vi "Robot Global Data.vi"() -> ()   [LabVIEW 2016]
doc: "This global VI can contain as many global variables as you need. Place a control on the panel, give it a good name. To read or write to it from a VI, drag the icon to the diagram of that VI. You can also drag from the project. Click on the node to change which global you access. You shouldn't have multiple locations writing to a global or it will cause a race-condition."
uses:
  <vilib>/Rock Robotics/WPI/Camera/WPI_CameraImageSize.ctl
  <vilib>/Rock Robotics/WPI/DriverStation/WPI_DriverStationRobotMode2.ctl
panel:
  out "Vision Nothing In Sight":bool
  in  "Autonoums Delay":dbl
  in  "Vision align Range correction VARIABLE":dbl
  in  "Vision align Oscillation correction VARIABLE":dbl
  in  "Autonomos Gyro forward SPEED VARIABLE":dbl
  in  "Periodic Gyro forward SPEED VARIABLE":dbl
  in  "Accelerometer Z Axis":dbl
  in  "Accelerometer Y Axis":dbl
  in  "Accelerometer X Axis":dbl
  out "Gyro Rest?":bool
  in  "LEFT SPEED VARIABLE":dbl
  out "Autonomous Operating":bool
  out "Vision needed":bool
  in  "RIGHT SPEED VARIABLE":dbl
  in  "ClimbMotors":dbl
  in  "Enum Teleop Control":u16
  in  "Enum Teleop":T1(ring)
  out "Teleop Operating":bool
  in  "String Teleop":string
  in  "Motor Array":dbl[](array[numeric])
  out "Vision Enabled":bool
  out "auto proceed":bool
  in  "Vision Turn":dbl
  in  "LeftMotors":dbl
  in  "RightMotors":dbl
  in  "X?":dbl
  out "In range?":bool
  out "Logitech Right 9":bool
  out "Logitech Left 9":bool
  out "Logitech Right 7":bool
  out "Logitech Right 5":bool
  out "Logitech Right 6":bool
  out "Logitech Right 8":bool
  out "Logitech Right 4":bool
  out "Logitech Right 3":bool
  out "Logitech Right 2":bool
  out "Logitech Right 1":bool
  out "Logitech Left 7":bool
  out "Logitech Left 5":bool
  out "Logitech Left 6":bool
  out "Logitech Left 8":bool
  out "Logitech Left 4":bool
  out "Logitech Left 3":bool
  out "Logitech Left 2":bool
  out "Logitech Left 1":bool
  in  "Logitech Right Slider":dbl
  in  "Logitech Right Z axis":dbl
  in  "Logitech Right Y axis":dbl
  in  "Logitech Right X axis":dbl
  in  "Logitech Left Slider":dbl
  in  "Logitech Left Z axis":dbl
  in  "Logitech Left Y axis":dbl
  in  "Logitech Left X axis":dbl
  out "Xbox Left Joystick Button":bool
  out "Xbox Back":bool
  out "Xbox LB":bool
  out "Xbox RB":bool
  out "Xbox Start":bool
  out "Xbox Y":bool
  out "Xbox X":bool
  out "Xbox B":bool
  out "Xbox A":bool
  in  "Xbox Left Trigger":dbl
  in  "Xbox Right Trigger":dbl
  in  "Xbox Right X axis":dbl
  in  "Xbox Right Y axis":dbl
  in  "Xbox Left X axis":dbl
  in  "Xbox Left Y axis":dbl
  in  "TopRightMotor":dbl
  in  "TopLeftMotor":dbl
  in  "GyroAngularRate":dbl
  in  "GyroAngle":dbl
  in  "Robot Mode":T2
  in  "image size":T3=enum."320x240"
  in  "Enable Vision":bool
  # "Power To Motors :"
  # "Accelerometer Axis Data"
  # "DASHBOARD VARIABLES"
  # "Vsion processing things"
  # "Motor Oversight"
  # "Turns on when Teleop is active"
  # "Gyro Data"
  # "Turns on when Autonomos is active"
  # "Logitech Joystick Right"
  # "Logitech Joystick Left"
  # "Xbox Controls :"
  # "Teleop controls"
  # "Dunno wut dis is"
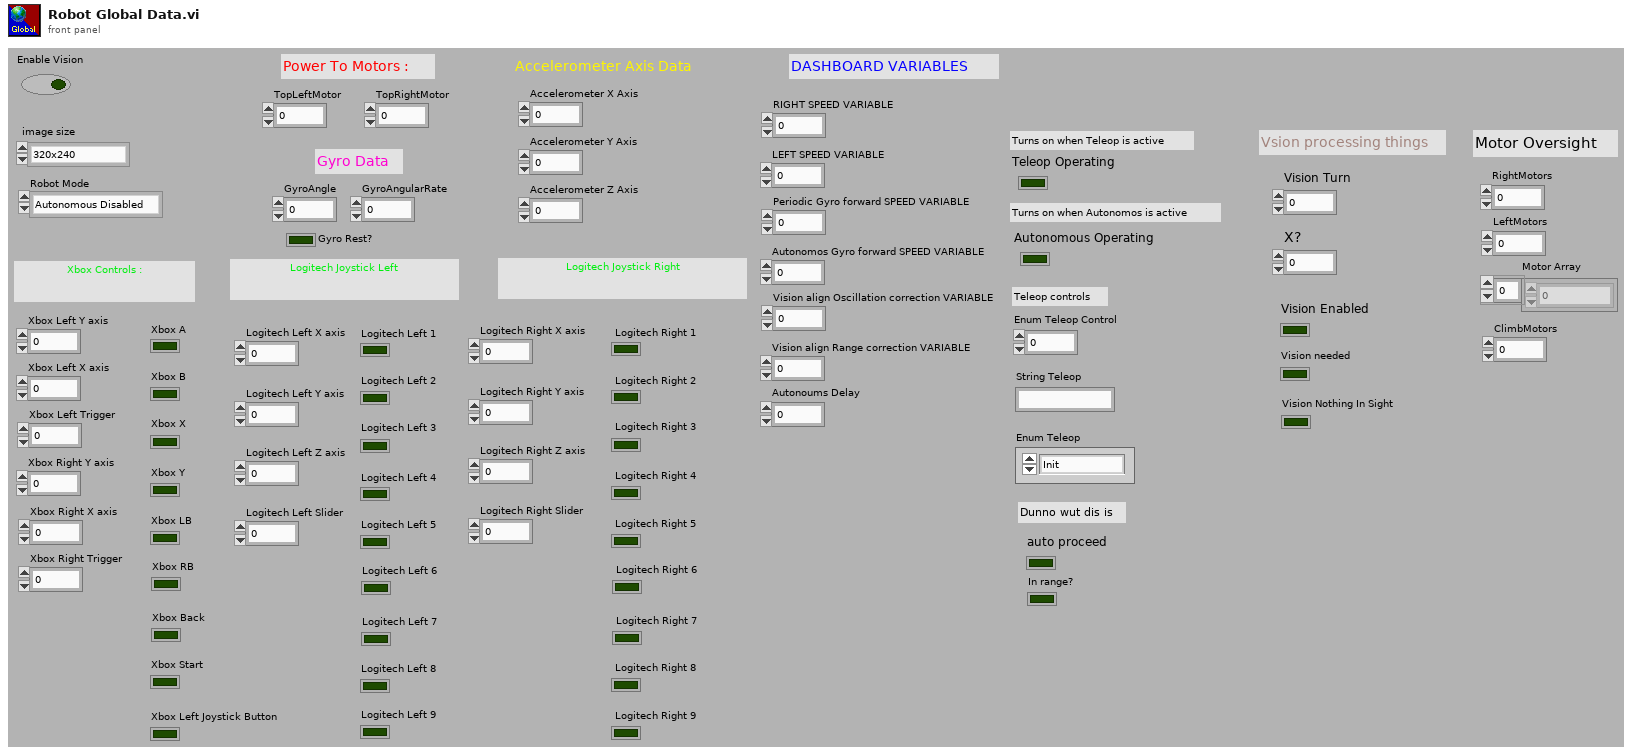
[diagram p1: front panel]
types:
  T1 = enum16{"Init", "Tank Motors", "Right Arcade", "Left Arcade", "Forward", "Back", "Vision Alignment", "Climb", "Stop"}
  T2 = typedef "WPI_DriverStationRobotMode2.ctl" = enum16{"Autonomous Disabled", "Autonomous Enabled", "Teleop Disabled", "Teleop Enabled", "Disconnected", "Finish", "Test Disabled", "Test Enabled", "Emergency Stopped"}
  T3 = typedef "WPI_CameraImageSize.ctl" = enum16{"640x480", "320x240", "160x120", "Custom"}
diagram:
